vi "draw a circle.vi"(5 "angular arc bounds":dbl=6.283185307179586, 6 "number of points":i32=20, 7 "angular arc center":dbl=3.141592653589793, 9 "center Y":dbl, 10 "center x":dbl, 11 "radius":dbl) -> (3 "output cluster":cluster{dbl[], dbl[]})   [LabVIEW 2018]
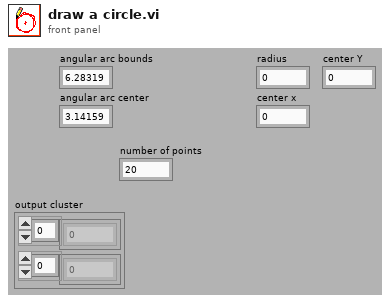
[diagram p1: front panel]
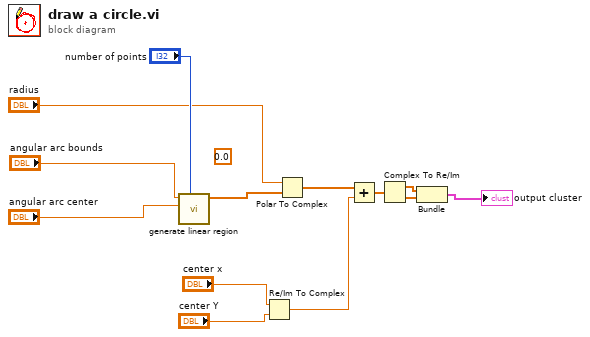
[diagram p0: block diagram]
diagram:
  (unwired) 0.0
  n1 = call "generate linear region.vi"("number of  grid points"="number of points", "center"="angular arc center", "delta"="angular arc bounds") -> ("real axis"=w2:dbl[])  [unwired: 8 in]
  n2 = Re/Im To Complex(1:"center Y", 2:"center x") -> (0:w4:cdb)
  n3 = Polar To Complex(1:w2, 2:"radius") -> (0:w1:cdb[])
  n4 = Add(x=w1, y=w4) -> (x+y=w13:cdb[])
  n5 = Complex To Re/Im(x + iy=w13) -> (x=w12:dbl[], y=w11:dbl[])
  n6 = Bundle(w12, w11) -> (→"output cluster":cluster{dbl[], dbl[]})  [unwired: 1 in]
